vi "New.vi"(8 "Error In":errorcluster, 11 "Key":string) -> (0 "Error Out":errorcluster, 3 "Begin Section":refnum<class "BeginSection.lvclass">)   [LabVIEW 2018, in "Toolkit.lvlib" / "Tokens.lvlib" / "BeginSection.lvclass"]
uses:
  BeginSection.lvclass
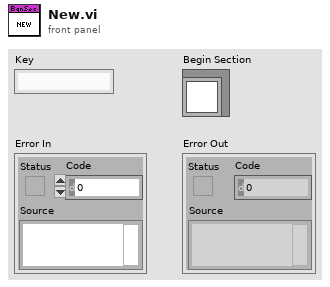
[diagram p1: front panel]
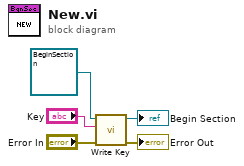
[diagram p0: block diagram]
diagram:
  n1 = call-dynamic "Write Key.vi"("Error In"="Error In", "Key"="Key", "Variable In"=refnum<class "BeginSection.lvclass"> refnum ("Mustache.lvlib:Tokens.lvlib:BeginSection.lvclass")) -> ("Error Out"=→"Error Out":errorcluster, "Variable Out"=→"Begin Section":refnum<class "BeginSection.lvclass">)  [unwired: 7 in]
